vi "CLStimSimple.vi"() -> ()   [LabVIEW 2017]
uses:
  <vilib>/DAQmx/write.llb/DAQmx Write (Analog Wfm 1Chan NSamp).vi
  <vilib>/DAQmx/read.llb/DAQmx Read (Counter U32 1Chan 1Samp).vi
  zmq_utilities/TTLReceive.vi
  <vilib>/DAQmx/miscellaneous.llb/DAQmx Fill In Error Info.vi
  <vilib>/addons/zeromq/zmq_recv_multi.vi
panel:
  in  "Sham stim channel":tag="pciDAQ/ao2"
  in  "Max add'l timeout \n(ms)":dbl=200.0
  in  "Sample rate":dbl=30000.0
  in  "Artifact padding\n (ms)":dbl=1000.0
  in  "OEP sample clock in":tag="/pciDAQ/PFI0"
  in  "Onboard counter":tag="pciDAQ/ctr0"
  in  "Real stim channel":tag="pciDAQ/ao0"
  out "Learning rate (for adaptive threshold)":dbl(graph)
  out "Phase threshold":sgl(graph)
  in  "Sham stimulations:":i32=1 min=0
  in  "Real stimulations:":i32=1 min=1
  out "Stim time":i64
  out "Crossing time":i64
  out "Crossing level":sgl
  out "Time on (samp.)":i64
  in  "Sham TTL chan":u16=3 caption="probe channel" min=1 max=8
  in  "Crossing TTL chan":u16=1 min=1 max=8
  in  "event port":u16=5557
  out "New event":bool
  in  "Stim enabled":bool
  out "OEP to LV delay":dbl(graph)
  in  "Stop":bool
  # "*** Start OpenEphys acquisition before the VI. ***"
  # "*** In the audio settings in the OpenEphys GUI, reduce the buffer size to get a 10 ms buffer period.  If ASIO is installed and enabled in\nthe Open Ephys build, use ASIO with sample rate (in audio settings) = 192,000 Hz and buffer size = 192 (1 ms buffer period). ***"
  # "Inputs"
  # "Event info"
  # "Timeout"
  # "Stim pattern if enabled"
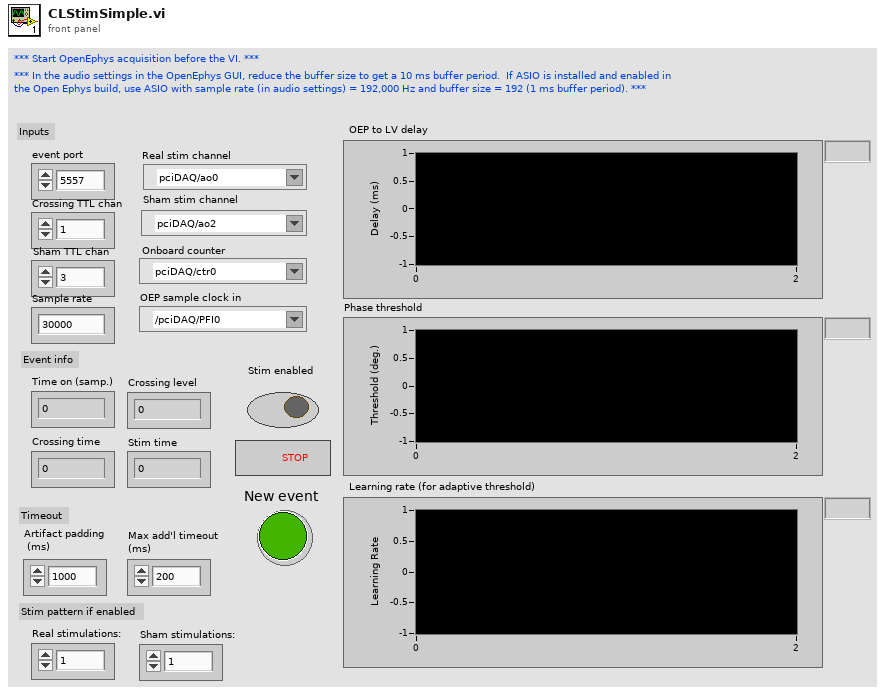
[diagram p1: front panel]
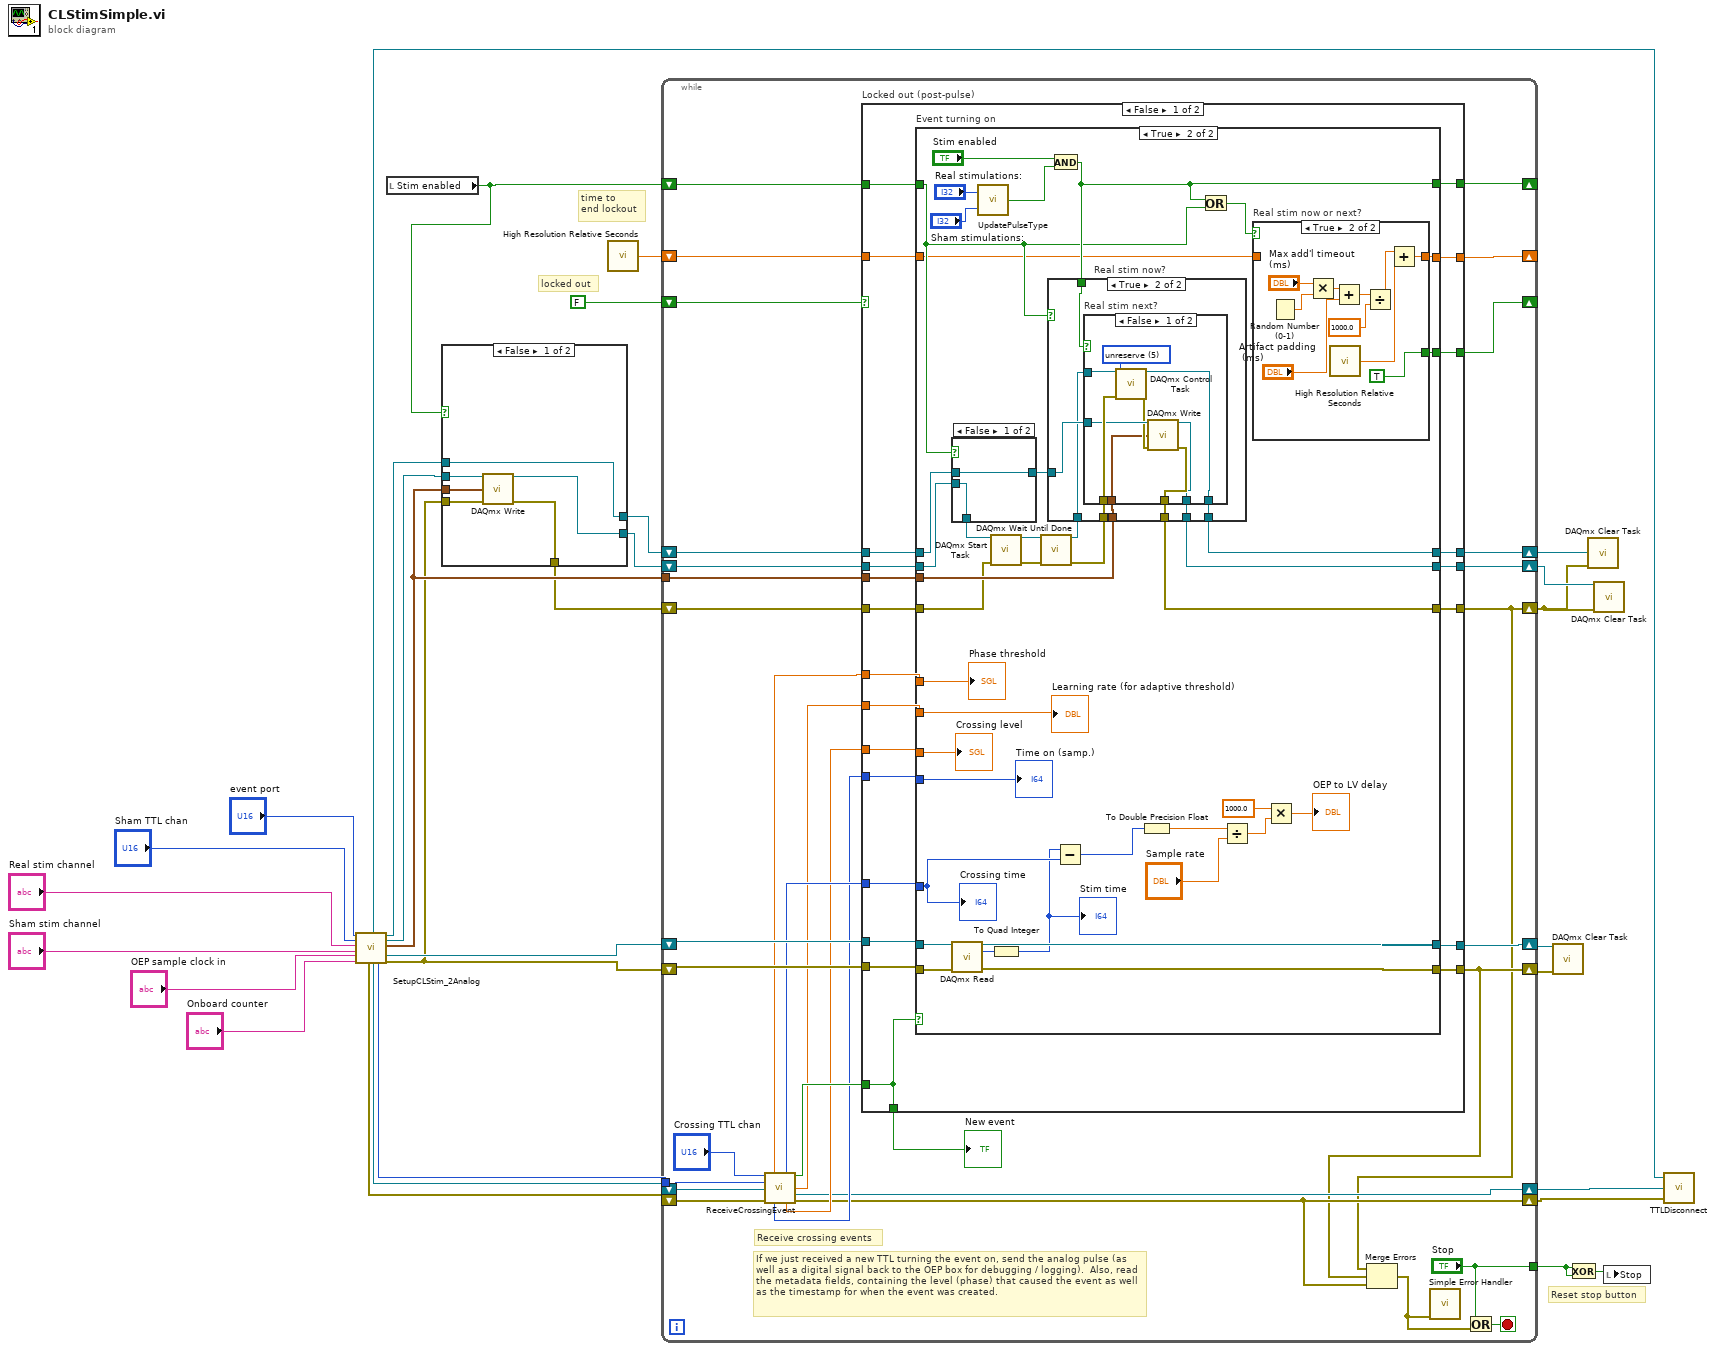
[diagram p0: block diagram]
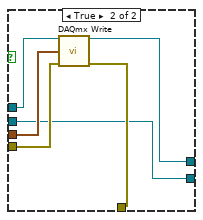
[diagram p2: hidden frame]
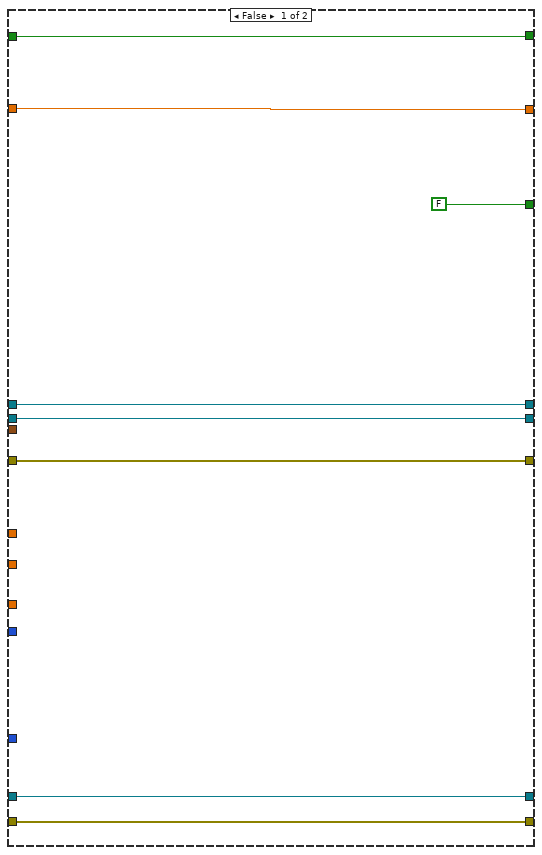
[diagram p3: hidden frame]
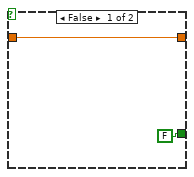
[diagram p4: hidden frame]
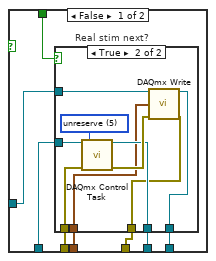
[diagram p6: hidden frame]
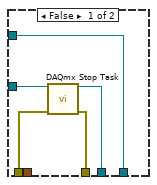
[diagram p7: hidden frame]
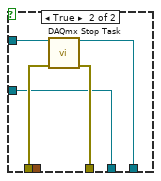
[diagram p8: hidden frame]
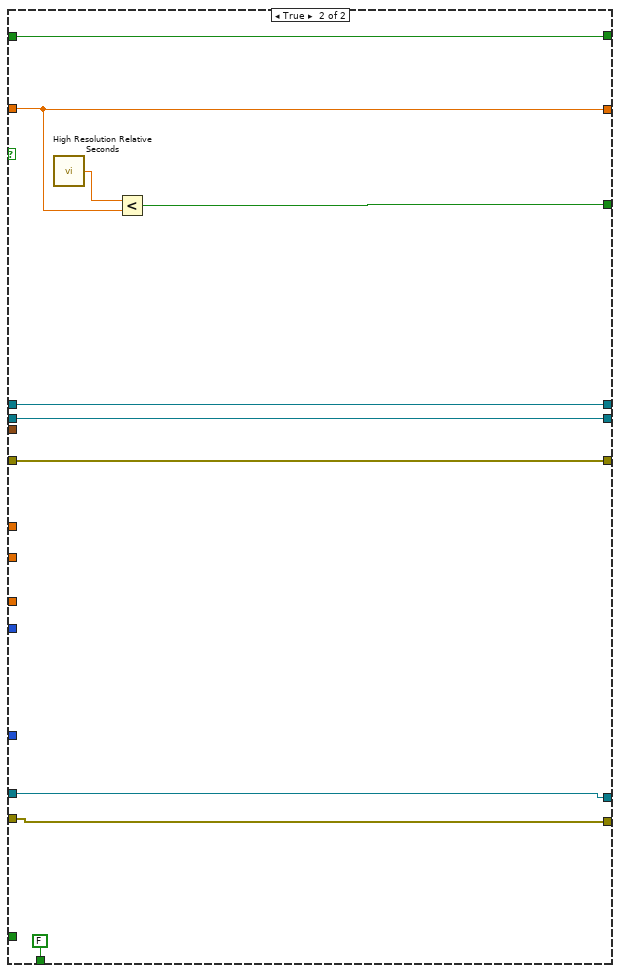
[diagram p9: hidden frame]
diagram:
  # "locked out"
  # "time to \nend lockout"
  # "Reset stop button"
  n1 = call "SetupCLStim_2Analog.vi"("event port"="event port", "Sham stim event channel"="Sham TTL chan", "Real stim channel"="Real stim channel", "Sham stim channel"="Sham stim channel", "OEP sample clock in"="OEP sample clock in", "Onboard counter"="Onboard counter") -> ("ZMQ error out"=w21:errorcluster, "context out"=w20:refnum<class "zmq_context.lvclass">, "socket out"=w22:refnum<class "zmq_socket.lvclass">, "clock offset"=w23:i64, "Real stim task"=w7:refnum<k21>, "Sham stim task"=w8:refnum<k21>, "Waveform Graph"=w6:waveform(dbl), "Ctr task"=w24:refnum<k21>, "DAQ error out"=w4:errorcluster)  [unwired: 5 in]
  n2 = local read "Stim enabled"() -> (w5:bool)
  n3 = case shown="False" w5 {
    tunnel: w8 -> [w34 w37]
    tunnel: w7 -> [w32 w41]
    tunnel: w6 -> [w35 w42]
    tunnel: w4 -> [w36 w40]
    tunnel: [w31 w39] -> w3
    tunnel: [w32 w38] -> w2
    tunnel: [w33 w37] -> w1
    frame False {
      n4 = call-poly <vilib>:"DAQmx Write.vi"("task/channels in"=w34, "data"=w35, "error in"=w36) -> ("task out"=w33:refnum<k21>, "error out"=w31:errorcluster)  [unwired: 10 in, 1 out]
    }
    frame True {
      n5 = call-poly <vilib>:"DAQmx Write.vi"("task/channels in"=w41, "data"=w42, "error in"=w40) -> ("task out"=w38:refnum<k21>, "error out"=w39:errorcluster)  [unwired: 10 in, 1 out]
    }
  }
  n6 = call <vilib>:"High Resolution Relative Seconds.vi"() -> ("relative seconds"=w16:dbl)
  n7 = while {
    tunnel: ["Stop"] -> w25
    shift-right: [w60] -> w11
    shift-left: w2 -> [w75]
    shift-right: [w45] -> w9
    shift-left: w3 -> [w73]
    shift-right: [w59] -> w29
    shift-left: w24 -> [w74]
    shift-right: [w55] -> w28
    shift-left: w4 -> [w72]
    shift-right: [w57] -> w27
    shift-left: w22 -> [w71]
    shift-right: [w56] -> w26
    shift-left: w21 -> [w70]
    tunnel: w23 -> [w54]
    shift-right: [w50] -> _
    shift-left: w16 -> [w49]
    shift-right: [w51] -> _
    shift-left: FALSE -> [w52]
    shift-right: [w47] -> w10
    shift-left: w1 -> [w48]
    tunnel: w6 -> [w46]
    shift-right: [w44] -> _
    shift-left: w5 -> [w43]
    stop <- w62 stop-if-true
    # "If we just received a new TTL turning the event on, send the analog pulse (as well as a digital signal back to the OEP box for debugging / logging).  Also, read the metadata fields, containing the level (phase) that caused the event as well as the timestamp for when the event was created."
    # "Receive crossing events"
    n8 = call "ReceiveCrossingEvent.vi"("channel"="Crossing TTL chan", "clock offset"=w54, "socket in"=w71, "error in"=w70) -> ("threshold"=w64:sgl, "new crossing"=w69:bool, "crossing time"=w68:i64, "learning rate"=w63:dbl, "socket out"=w57:refnum<class "zmq_socket.lvclass">, "event time"=w67:i64, "crossing level"=w66:sgl, "error out"=w56:errorcluster)  [unwired: 3 in, 1 out]
    n9 = case "Locked out (post-pulse)" shown="False" w52 {
      tunnel: w75 -> [w97 w212]
      tunnel: w74 -> [w96 w213]
      tunnel: w73 -> [w95 w211]
      tunnel: w72 -> [w94 w214]
      tunnel: w69 -> [w84 _]
      tunnel: w68 -> [w93 _]
      tunnel: w67 -> [w92 _]
      tunnel: w66 -> [w91 _]
      tunnel: w64 -> [w90 _]
      tunnel: w63 -> [w89 _]
      tunnel: [w88 w212] -> w60
      tunnel: [w87 w213] -> w59
      tunnel: [w86 w211] -> w45
      tunnel: [w85 w214] -> w55
      tunnel: [w84 FALSE ("new crossing")] -> w53
      tunnel: [w82 w208] -> w51
      tunnel: [w81 w210] -> w50
      tunnel: w49 -> [w83 w210]
      tunnel: w48 -> [w80 w207]
      tunnel: [w79 w207] -> w47
      tunnel: w46 -> [w78 _]
      tunnel: [w77 w206] -> w44
      tunnel: w43 -> [w76 w206]
      frame False {
        n10 = case "Event turning on" shown="True" w84 {
          tunnel: w97 -> [w105 w120]
          tunnel: w95 -> [w104 w123]
          tunnel: [w105 w114] -> w88
          tunnel: [w104 w113] -> w86
          tunnel: w93 -> [_ w139]
          tunnel: w96 -> [w103 w145]
          tunnel: w94 -> [w102 w143]
          tunnel: [w103 w142] -> w87
          tunnel: [w102 w141] -> w85
          tunnel: w92 -> [_ w140]
          tunnel: w91 -> [_ w138]
          tunnel: w90 -> [_ w137]
          tunnel: w89 -> [_ w136]
          tunnel: [w101 w107] -> w81
          tunnel: w83 -> [w101 w106]
          tunnel: [FALSE w108] -> w82
          tunnel: w80 -> [w99 w119]
          tunnel: [w99 w112] -> w79
          tunnel: w78 -> [_ w124]
          tunnel: [w98 w110] -> w77
          tunnel: w76 -> [w98 w109]
          frame False {
          }
          frame True {
            n11 = case shown="False" w109 {
              tunnel: w120 -> [w158 w161]
              tunnel: w119 -> [w159 w160]
              tunnel: [w159 w161] -> w118
              tunnel: [w158 w160] -> w117
              frame False {
              }
              frame True {
              }
            }
            n12 = call-poly <vilib>:"DAQmx Read.vi"("task/channels in"=w145, "error in"=w143) -> ("task out"=w142:refnum<k21>, "data"=w144:u32, "error out"=w141:errorcluster)  [unwired: 11 in]
            n13 = call "UpdatePulseType.vi"("Sham stimulations:"="Sham stimulations:", "Real stimulations:"="Real stimulations:") -> ("Real stim on"=w125:bool)
            n14 = call <vilib>:"DAQmx Start Task.vi"("task/channels in"=w118, "error in"=w123) -> ("task out"=w122:refnum<k21>, "error out"=w121:errorcluster)  [unwired: 12 in]
            n15 = To Quad Integer(1:w144) -> (0:w135:i64)
            "Stim time" <- w135
            n16 = call <vilib>:"DAQmx Wait Until Done.vi"("task/channels in"=w122, "error in"=w121) -> ("task out"=w116:refnum<k21>, "error out"=w115:errorcluster)  [unwired: 12 in]
            n17 = And(x="Stim enabled", y=w125) -> (x .and. y?=w110:bool)
            n18 = case "Real stim now?" shown="True" w109 {
              tunnel: w110 -> [w169 w191]
              tunnel: w124 -> [w162 w190]
              tunnel: w117 -> [w168 w189]
              tunnel: w116 -> [w167 w188]
              tunnel: w115 -> [w166 w187]
              tunnel: [w163 w186] -> w114
              tunnel: [w165 w185] -> w113
              tunnel: [w164 w184] -> w112
              frame False {
                n19 = case "Real stim next?" shown="True" w169 {
                  tunnel: w168 -> [w170 w178]
                  tunnel: w167 -> [w174 w183]
                  tunnel: w166 -> [w173 w182]
                  tunnel: [w172 w177] -> w165
                  tunnel: [w171 w179] -> w164
                  tunnel: [w170 w176] -> w163
                  tunnel: w162 -> [_ w175]
                  frame False {
                    n20 = call <vilib>:"DAQmx Stop Task.vi"("task/channels in"=w174, "error in"=w173) -> ("task out"=w171:refnum<k21>, "error out"=w172:errorcluster)  [unwired: 12 in]
                  }
                  frame True {
                    w181 = 5 items=["verify"=2, "reserve"=4, "commit"=3, "unreserve"=5, "abort"=6] ("action")
                    n21 = call <vilib>:"DAQmx Control Task.vi"("task/channels in"=w183, "action"=w181, "error in"=w182) -> ("task out"=w179:refnum<k21>, "error out"=w180:errorcluster)  [unwired: 11 in]
                    n22 = call-poly <vilib>:"DAQmx Write.vi"("task/channels in"=w178, "data"=w175, "error in"=w180) -> ("task out"=w176:refnum<k21>, "error out"=w177:errorcluster)  [unwired: 10 in, 1 out]
                  }
                }
              }
              frame True {
                n23 = case "Real stim next?" shown="False" w191 {
                  tunnel: w190 -> [w195 _]
                  tunnel: w189 -> [w197 w202]
                  tunnel: w188 -> [w200 w205]
                  tunnel: w187 -> [w198 w204]
                  tunnel: [w194 w201] -> w186
                  tunnel: [w193 w203] -> w185
                  tunnel: [w192 w202] -> w184
                  frame False {
                    w199 = 5 items=["verify"=2, "reserve"=4, "commit"=3, "unreserve"=5, "abort"=6] ("action")
                    n24 = call <vilib>:"DAQmx Control Task.vi"("task/channels in"=w200, "action"=w199, "error in"=w198) -> ("task out"=w194:refnum<k21>, "error out"=w196:errorcluster)  [unwired: 11 in]
                    n25 = call-poly <vilib>:"DAQmx Write.vi"("task/channels in"=w197, "data"=w195, "error in"=w196) -> ("task out"=w192:refnum<k21>, "error out"=w193:errorcluster)  [unwired: 10 in, 1 out]
                  }
                  frame True {
                    n26 = call <vilib>:"DAQmx Stop Task.vi"("task/channels in"=w205, "error in"=w204) -> ("task out"=w201:refnum<k21>, "error out"=w203:errorcluster)  [unwired: 12 in]
                  }
                }
              }
            }
            n27 = Subtract(x=w135, y=w139) -> (x-y=w130:i64)
            n28 = To Double Precision Float(number=w130) -> (double precision float=w132:dbl)
            n29 = Or(x=w110, y=w109) -> (x .or. y?=w111:bool)
            n30 = Divide(x=w132, y="Sample rate") -> (x/y=w128:dbl)
            n31 = case "Real stim now or next?" shown="True" w111 {
              tunnel: [FALSE TRUE] -> w108
              tunnel: [w146 w148] -> w107
              tunnel: w106 -> [w146 _]
              frame False {
              }
              frame True {
                n32 = Random Number (0-1)() -> (number: 0 to 1=w157:dbl)
                n33 = Multiply(x="Max add'l timeout \n(ms)", y=w157) -> (x*y=w153:dbl)
                n34 = call <vilib>:"High Resolution Relative Seconds.vi"() -> ("relative seconds"=w151:dbl)
                n35 = Add(x=w153, y="Artifact padding\n (ms)") -> (x+y=w154:dbl)
                n36 = Divide(x=w154, y=1000.0) -> (x/y=w155:dbl)
                n37 = Add(x=w155, y=w151) -> (x+y=w148:dbl)
              }
            }
            n38 = Multiply(x=1000.0, y=w128) -> (x*y=→"OEP to LV delay":dbl)
            "Time on (samp.)" <- w140
            "Crossing time" <- w139
            "Crossing level" <- w138
            "Phase threshold" <- w137
            "Learning rate (for adaptive threshold)" <- w136
          }
        }
      }
      frame True {
        n39 = call <vilib>:"High Resolution Relative Seconds.vi"() -> ("relative seconds"=w209:dbl)
        n40 = Less?(x=w209, y=w210) -> (x < y?=w208:bool)
      }
    }
    "New event" <- w53
    n41 = Merge Errors(w45, w55, w56) -> (w58:errorcluster)
    n42 = call <vilib>:"Simple Error Handler.vi"("error in (no error)"=w58) -> ()  [unwired: 4 in, 5 out]
    n43 = Or(x="Stop", y=w58) -> (x .or. y?=w62:bool)
  }
  n44 = call <vilib>:"DAQmx Clear Task.vi"("task in"=w29, "error in"=w28) -> ()  [unwired: 13 in, 1 out]
  n45 = Exclusive Or(1:w25, 2:w25) -> (0:w30:bool)
  n46 = call <vilib>:"DAQmx Clear Task.vi"("task in"=w11, "error in"=w9) -> ()  [unwired: 13 in, 1 out]
  n47 = call <vilib>:"DAQmx Clear Task.vi"("task in"=w10, "error in"=w9) -> ()  [unwired: 13 in, 1 out]
  n48 = local write "Stop"(w30) -> ()
  n49 = call "TTLDisconnect.vi"("error in"=w26, "socket in"=w27, "context in"=w20) -> ()  [unwired: 1 in, 1 out]
